vi "lsl push sample.vi"   [LabVIEW 2018, in "liblsl-LabVIEW.lvlib"]
uses:
  <userlib>/liblsl-LabVIEW/liblsl-LabVIEW.lvlib
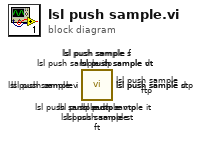
[diagram p0: block diagram]
diagram:
  n1 = call <userlib>:"lsl push sample vtp.vi"() -> ()  [unwired: 10 in, 2 out]
  n2 = call <userlib>:"lsl push sample vt.vi"() -> ()  [unwired: 10 in, 2 out]
  n3 = call <userlib>:"lsl push sample v.vi"() -> ()  [unwired: 10 in, 2 out]
  n4 = call <userlib>:"lsl push sample stp.vi"() -> ()  [unwired: 10 in, 2 out]
  n5 = call <userlib>:"lsl push sample st.vi"() -> ()  [unwired: 10 in, 2 out]
  n6 = call <userlib>:"lsl push sample s.vi"() -> ()  [unwired: 10 in, 2 out]
  n7 = call <userlib>:"lsl push sample itp.vi"() -> ()  [unwired: 10 in, 2 out]
  n8 = call <userlib>:"lsl push sample it.vi"() -> ()  [unwired: 10 in, 2 out]
  n9 = call <userlib>:"lsl push sample i.vi"() -> ()  [unwired: 10 in, 2 out]
  n10 = call <userlib>:"lsl push sample ftp.vi"() -> ()  [unwired: 10 in, 2 out]
  n11 = call <userlib>:"lsl push sample ft.vi"() -> ()  [unwired: 10 in, 2 out]
  n12 = call <userlib>:"lsl push sample f.vi"() -> ()  [unwired: 10 in, 2 out]
  n13 = call <userlib>:"lsl push sample dtp.vi"() -> ()  [unwired: 10 in, 2 out]
  n14 = call <userlib>:"lsl push sample dt.vi"() -> ()  [unwired: 10 in, 2 out]
  n15 = call <userlib>:"lsl push sample d.vi"() -> ()  [unwired: 10 in, 2 out]
